vi "closeGlobalFileRef.vi"   [LabVIEW 2010]
uses:
  AmmeterGlobalCostants.vi
  <vilib>/xml/Close Reference(Node).vi
  <vilib>/xml/NI_XML.lvlib
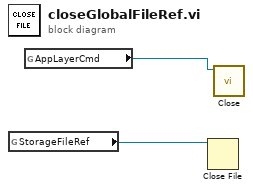
[diagram p0: block diagram]
diagram:
  n1 = global read "AmmeterGlobalCostants.vi" "StorageFileRef"() -> (w2:refnum<file>)
  n2 = global read "AmmeterGlobalCostants.vi" "AppLayerCmd"() -> (w1:refnum<k20>)
  n3 = Close File(refnum=w2) -> ()  [unwired: 1 in, 2 out]
  n4 = call-poly <vilib>:"Close.vi"("node"=w1) -> ()  [unwired: 8 in, 1 out]
